vi "GenerateChangedLibrariesList.vi"(6 "GUI Mode? {F)":bool, 8 "error in (no error)":errorcluster, 11 "Workspace Path":path=path "E:/sw-deps-monitor") -> (0 "error out":errorcluster)   [LabVIEW 2023, in "DepsWatch.lvlib"]
uses:
  DepsWatch.lvlib
  ead0c1dc-4abe-4fdf-93af-0a2c3e7fff4b.vi
  <vilib>/Wiresmith Technology/G CLI/CLI Class/CLI.lvclass
panel:
  in  "Tab Control":enum32{"GUI Mode", "CLI Mode"}(tab)=enum."CLI Mode"
  out "Args":string[](array[string])=["E:\\sw-deps-monitor"]
  # "When in GUI Mode, the controls will be used, \nin CLI Mode the Args will be used"
  # "Command to run the VI from terminal\n\ng-cli -v --lv-ver 2023 --arch 32 \"E:\\sw-deps-monitor\\CICD\\CheckModifiedVIs\\GenerateChangedLibrariesList.vi\" -- \"E:\\sw-deps-monitor\""
  # "Workspace Path"
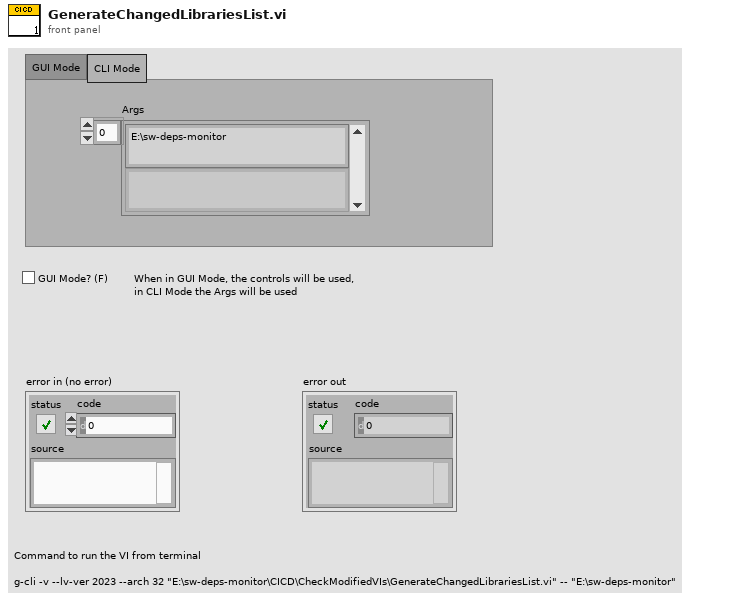
[diagram p1: front panel]
types:
  T1 = enum16{"open", "replace", "create", "open or create", "replace or create", "replace or create with confirmation"}
  T2 = typedef "DepsWatch.lvlib/CICDPathConfigs.ctl" = cluster{"GlobalIncludePaths":path[], "GlobalExcludePaths":path[], "BuildSpecsIncludePaths":path[], "ActualDepsIncludePaths":path[], "WorkspacePath":path, "SourceFolderPaths":path[], "ChangedFilesLogpaths":map{string, path}}
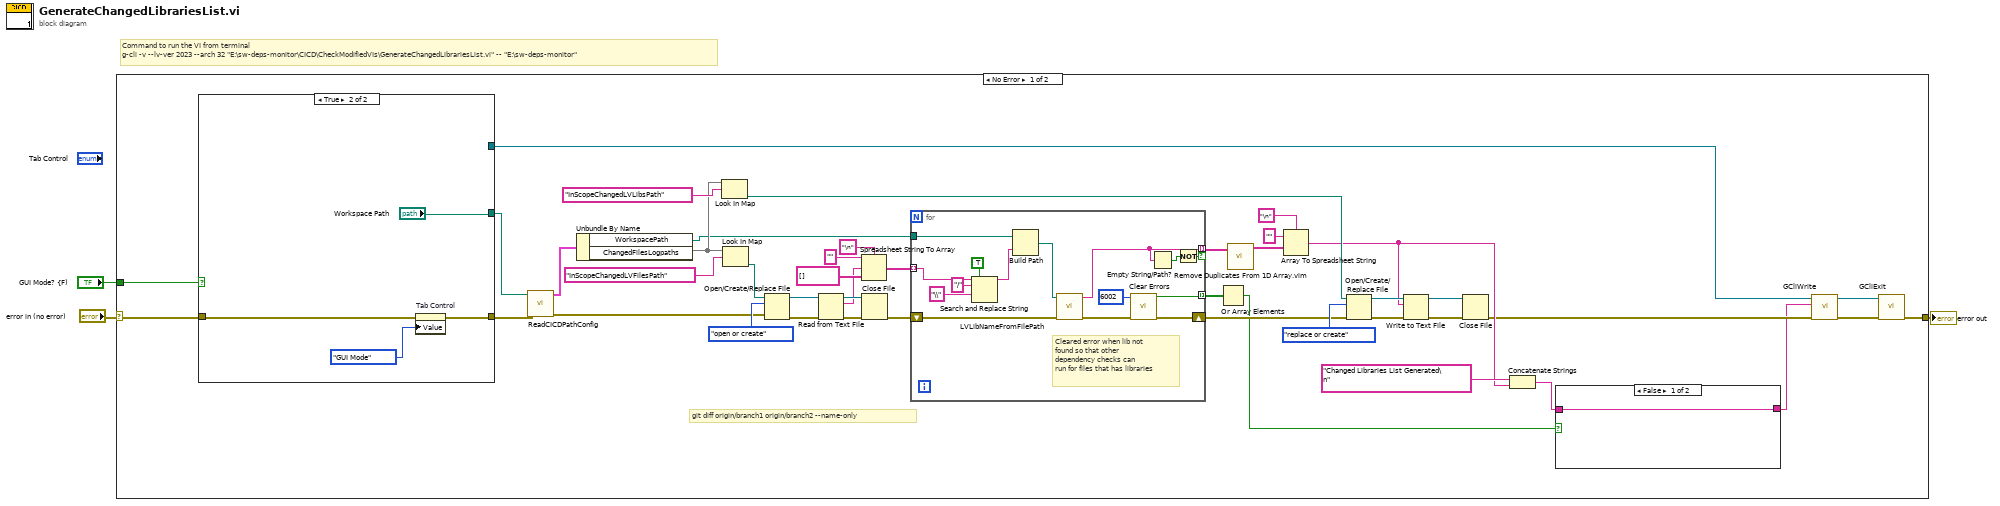
[diagram p0: block diagram]
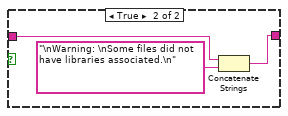
[diagram p2: hidden frame]
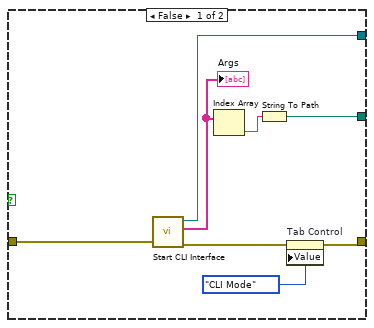
[diagram p3: hidden frame]
diagram:
  # "Command to run the VI from terminal\ng-cli -v --lv-ver 2023 --arch 32 \"E:\\sw-deps-monitor\\CICD\\CheckModifiedVIs\\GenerateChangedLibrariesList.vi\" -- \"E:\\sw-deps-monitor\""
  n1 = case shown="No Error" "error in (no error)" {
    selector: "error in (no error)" -> [w46 w79]
    tunnel: "GUI Mode? {F)" -> [w47 _]
    tunnel: [w42 w79] -> w1
    frame No Error {
      # "git diff origin/branch1 origin/branch2 --name-only"
      n2 = case shown="True" w47 {
        tunnel: [w73 "Workspace Path"] -> w39
        tunnel: w46 -> [w72 w77]
        tunnel: [w70 w75] -> w38
        tunnel: [w71 _] -> w44
        frame False {
          n3 = call <vilib>:"Start CLI Interface.vi"("error in (no error)"=w72) -> ("error out"=w68:errorcluster, "Custom Parameters"=w67:string[], "CLI out"=w71:refnum<class "CLI.lvclass">)  [unwired: 7 in, 1 out]
          "Args" <- w67
          n4 = Index Array(array=w67) -> (element=w74:string)  [unwired: 1 in]
          n5 = String To Path(string=w74) -> (path=w73:path)
          n6 = property on="Tab Control" class="TabCtl (strict)"(error in=w68, "Value"=enum32{"GUI Mode", "CLI Mode"}."CLI Mode" ("Tab Control")) -> (error out=w70:errorcluster)  [unwired: 1 in, 1 out]
        }
        frame True {
          n7 = property on="Tab Control" class="TabCtl (strict)"(error in=w77, "Value"=enum32{"GUI Mode", "CLI Mode"}."GUI Mode" ("Tab Control")) -> (error out=w75:errorcluster)  [unwired: 1 in, 1 out]
        }
      }
      n8 = call "ReadCICDPathConfig.vi"("error in (no error)"=w38, "Workspace Path"=w39) -> ("error out"=w27:errorcluster, "CICD Path Config Out"=w37:T2)  [unwired: 8 in]
      n9 = Unbundle By Name(w37) -> ("WorkspacePath"=w17:path, "ChangedFilesLogpaths"=w25:map{string, path})
      n10 = Look In Map(map=w25, key="InScopeChangedLVLibsPath") -> (value=w24:path)  [unwired: 1 in, 1 out]
      n11 = Look In Map(map=w25, key="InScopeChangedLVFilesPath") -> (value=w35:path)  [unwired: 1 in, 1 out]
      n12 = Open/Create/Replace File(file path (use dialog)=w35, error in=w27, operation (0:open)=T1."open or create") -> (refnum out=w34:refnum<file>, error out=w33:errorcluster)  [unwired: 3 in, 1 out]
      n13 = Read from Text File(file (use dialog)=w34, error in=w33) -> (refnum out=w32:refnum<file>, text=w29:string, error out=w31:errorcluster)  [unwired: 2 in, 1 out]
      n14 = Spreadsheet String To Array(delimiter (Tab)="\n", format string="", spreadsheet string=w29, array type (2D Dbl)=string[] []) -> (array=w18:string[])
      n15 = Close File(refnum=w32, error in=w31) -> (error out=w16:errorcluster)  [unwired: 1 out]
      n16 = for {
        tunnel: w18 -> [w62] mode=indexing
        tunnel: w17 -> [w66]
        tunnel: [w55] -> w9 mode=indexing if=w53
        shift-right: [w57] -> w13
        shift-left: w16 -> [w65]
        tunnel: [w52] -> w7 mode=indexing
        # "Cleared error when lib not\nfound so that other\ndependency checks can\nrun for files that has libraries"
        n17 = Search and Replace String(replace all?=TRUE ("replace all? (F)"), input string=w62, search string="/", replace string="\\" ("replace string (\"\")")) -> (result string=w58:string)  [unwired: 4 in, 3 out]
        n18 = Build Path(base path=w66, name or relative path=w58) -> (appended path=w64:path)
        n19 = call "LVLibNameFromFilePath.vi"("error in (no error)"=w65, "LV File Path"=w64) -> ("error out"=w63:errorcluster, "Library Name"=w55:string)  [unwired: 8 in]
        n20 = call <vilib>:"Clear Errors.vi"("error in (no error)"=w63, "specific error code to clear (0: all)"=6002) -> ("error out"=w57:errorcluster, "specific error cleared?"=w52:bool)  [unwired: 4 in]
        n21 = Empty String/Path?(string/path=w55) -> (empty?=w54:bool)
        n22 = Not(x=w54) -> (.not. x?=w53:bool)
      }
      n23 = Or Array Elements(Boolean array=w7) -> (logical OR=w5:bool)
      n24 = call "Remove Duplicates From 1D Array.vim"("array"=w9) -> ("array with duplicates removed"=w8:string[])  [unwired: 10 in]
      n25 = Array To Spreadsheet String(delimiter (Tab)="\n", array=w8, 3:"" ("format string")) -> (spreadsheet string=w12:string)
      n26 = Open/Create/Replace File(file path (use dialog)=w24, error in=w13, operation (0:open)=T1."replace or create") -> (refnum out=w21:refnum<file>, error out=w22:errorcluster)  [unwired: 3 in, 1 out]
      n27 = Write to Text File(file (use dialog)=w21, text=w12, error in=w22) -> (refnum out=w19:refnum<file>, error out=w20:errorcluster)  [unwired: 1 in, 1 out]
      n28 = Close File(refnum=w19, error in=w20) -> (error out=w11:errorcluster)  [unwired: 1 out]
      n29 = Concatenate Strings("Changed Libraries List Generated\n" ("Text to Write"), w12) -> (w6:string)
      n30 = case shown="False" w5 {
        tunnel: w6 -> [w48 w51]
        tunnel: [w48 w49] -> w4
        frame False {
        }
        frame True {
          n31 = Concatenate Strings(w51, "\nWarning: \nSome files did not have libraries associated.\n" ("Text to Write")) -> (w49:string)
        }
      }
      n32 = call "GCliWrite.vi"("error in (no error)"=w11, "Text to Write"=w4, "CLI in"=w44) -> ("error out"=w43:errorcluster, "CLI out"=w41:refnum<class "CLI.lvclass">)  [unwired: 7 in]
      n33 = call "GCliExit.vi"("error in (no error)"=w43, "CLI in"=w41) -> ("error out"=w42:errorcluster)  [unwired: 9 in]
    }
    frame Error {
    }
  }
  "error out" <- w1
